vi "Software Update HCC Change INI File.vi"(8 "Error In":errorcluster, 10 "Array":path[](array[path])) -> (0 "Error Out":errorcluster)   [LabVIEW 2016]
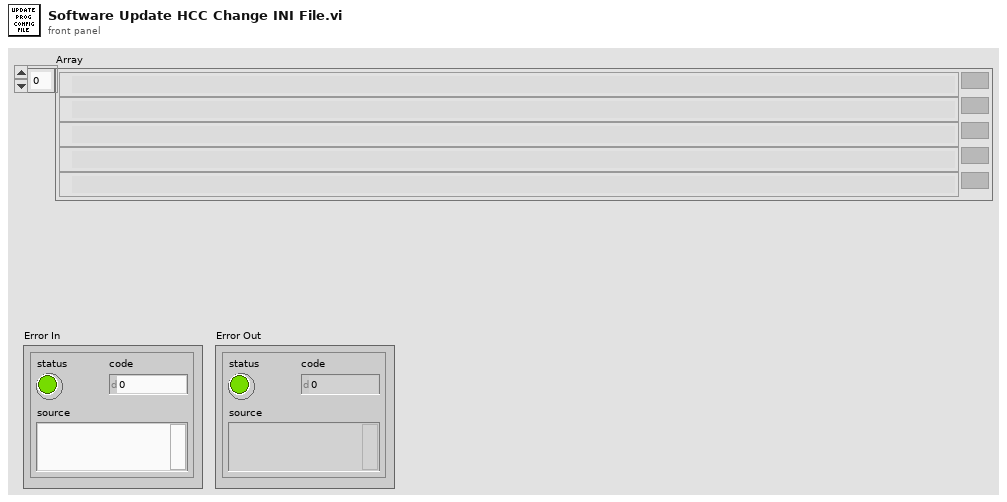
[diagram p1: front panel]
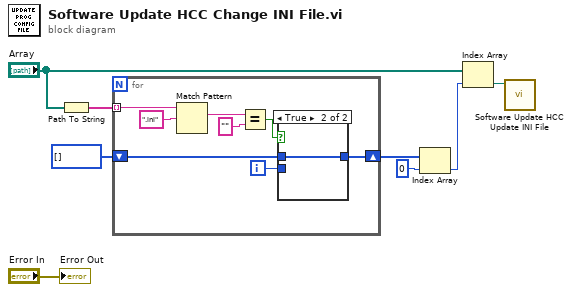
[diagram p0: block diagram]
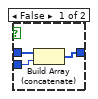
[diagram p2: hidden frame]
diagram:
  n1 = Path To String(path="Array") -> (string=w5:string[])
  n2 = for {
    tunnel: w5 -> [w16] mode=indexing
    shift-right: [w10] -> w7
    shift-left: i32[] [] -> [w11]
    i -> [w9]
    n3 = Match Pattern(string=w16, regular expression=".ini") -> (match substring=w14:string)  [unwired: 1 in, 3 out]
    n4 = Equal?(x=w14, y="") -> (x = y?=w12:bool)
    n5 = case shown="True" w12 {
      tunnel: w11 -> [w19 w20]
      tunnel: [w18 w20] -> w10
      tunnel: w9 -> [w17 _]
      frame False {
        n6 = Build Array (concatenate)(w19, w17) -> (w18:i32[])
      }
      frame True {
      }
    }
  }
  n7 = Index Array(array=w7, index=0) -> (element=w3:i32)
  n8 = Index Array(array="Array", index=w3) -> (element=w2:path)
  n9 = call "Software Update HCC Update INI File.vi"("Path"=w2) -> ()  [unwired: 11 in]
  "Error Out" <- "Error In"
